vi "Read Support RFC3339.vi"(11 "DateTime.ISO8601 in":refnum<class "DateTime.ISO8601.lvclass">) -> (2 "Support RFC3339":bool=TRUE, 3 "DateTime.ISO8601 out":refnum<class "DateTime.ISO8601.lvclass">)   [LabVIEW 2018, in "DateTime.ISO8601.lvclass"]
uses:
  DateTime.ISO8601.lvclass
  DateTime.ISO8601.lvclass/DateTime.ISO8601.ctl
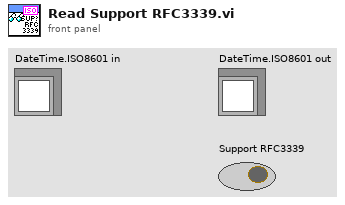
[diagram p1: front panel]
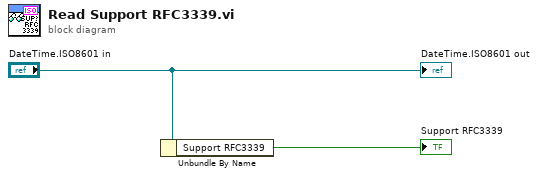
[diagram p0: block diagram]
diagram:
  n1 = Unbundle By Name("DateTime.ISO8601 in") -> ("Support RFC3339"=→"Support RFC3339":bool)
  "DateTime.ISO8601 out" <- "DateTime.ISO8601 in"
